vi "Fit T1.vi"(11 "XY Graph in":cluster{dbl[], dbl[]}[](graph)) -> (2 "T1 Fit Result":T1 {"T1" format="%#_6p"}, 3 "XY Graph out":cluster{dbl[], dbl[]}[](graph))   [LabVIEW 2020]
uses:
  <vilib>/Analysis/6fits.llb/Curve Fitting Criteria.ctl
  <vilib>/Analysis/NI_AALPro.lvlib
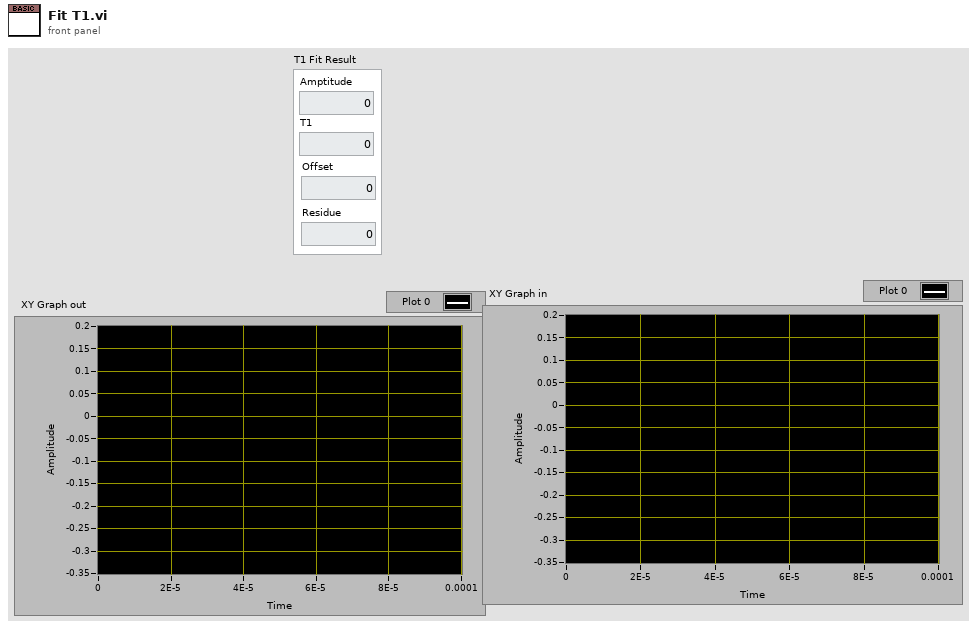
[diagram p1: front panel]
types:
  T1 = cluster{"Amptitude":dbl, "T1":dbl, "Offset":dbl, "Residue":dbl}
  T2 = typedef "NI_AALPro.lvlib/Curve Fitting Criteria.ctl" = u16
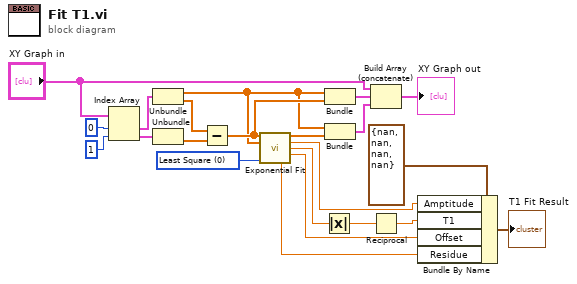
[diagram p0: block diagram]
diagram:
  w13 = T2 0 items=["Least Square", "Least Absolute Residual", "Bisquare"] ("method")
  n1 = Index Array(array="XY Graph in", index #1=0 ("index"), index #2=1 ("index")) -> (element #1=w20:cluster{dbl[], dbl[]}, element #2=w19:cluster{dbl[], dbl[]})
  n2 = Unbundle(w20) -> (w12:dbl[], w18:dbl[])
  n3 = Unbundle(w19) -> (w17:dbl[])  [unwired: 1 out]
  n4 = Subtract(x=w18, y=w17) -> (x-y=w14:dbl[])
  n5 = call <vilib>:"Exponential Fit.vi"("Y"=w14, "X"=w12, "method"=w13) -> ("Best Exponential Fit"=w11:dbl[], "amplitude"=w4:dbl, "damping"=w9:dbl, "offset"=w3:dbl, "residue"=w2:dbl)  [unwired: 7 in, 1 out]
  n6 = Absolute Value(x=w9) -> (abs(x)=w8:dbl)
  n7 = Bundle(w12, w14) -> (w16:cluster{dbl[], dbl[]})  [unwired: 1 in]
  n8 = Bundle(w12, "Best Exponential Fit"=w11) -> (w10:cluster{dbl[], "Best Exponential Fit":dbl[]})  [unwired: 1 in]
  n9 = Build Array (concatenate)("XY Graph in", w16, w10) -> (→"XY Graph out":cluster{dbl[], "Best Exponential Fit":dbl[]}[])
  n10 = Reciprocal(x=w8) -> (1/x=w5:dbl)
  n11 = Bundle By Name(cluster=T1 {"Amptitude"=nan, "T1"=nan, "Offset"=nan, "Residue"=nan} ("T1 Fit Result"), "Amptitude"=w4, "T1"=w5, "Offset"=w3, "Residue"=w2) -> (→"T1 Fit Result":T1)
